vi "LJStreamM default register list.vi"() -> (0 "Default Register List":string[](array[string])=["DAC0", "DAC1", "AIN_ALL_RESOLUTION_INDEX", "AIN_ALL_RANGE", "AIN0_NEGATIVE_CH", "AIN0_EF_INDEX", "AIN0_EF_CONFIG_A", "DIO4_EF_INDEX", "DIO4_EF_CONFIG_A", "DIO4_EF_ENABLE"])   [LabVIEW 2026]
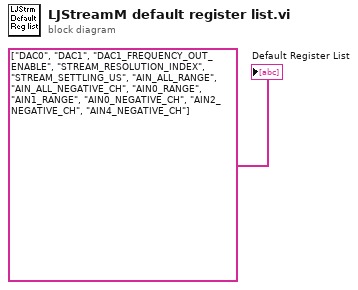
[diagram p0: block diagram]
diagram:
  "Default Register List" <- string[] ["DAC0", "DAC1", "DAC1_FREQUENCY_OUT_ENABLE", "STREAM_RESOLUTION_INDEX", "STREAM_SETTLING_US", "AIN_ALL_RANGE", "AIN_ALL_NEGATIVE_CH", "AIN0_RANGE", "AIN1_RANGE", "AIN0_NEGATIVE_CH", "AIN2_NEGATIVE_CH", "AIN4_NEGATIVE_CH"]
